vi "Register Message Metadata.vi"(8 "error in (no error)":errorcluster, 10 "Messages":T2[](array[typedef]), 11 "gRPCid":T1) -> (0 "error out":errorcluster, 3 "gRPCid":T1)   [LabVIEW 2020, in "helloWServer.lvlib" / "gprc-lvsupport.lvlib"]
uses:
  gprc-lvsupport.lvlib
  typeDefs/Message Metadata.ctl
  typeDefs/Message Element Metadata.ctl
  typeDefs/Message Element Type.ctl
  typeDefs/grpcId.ctl
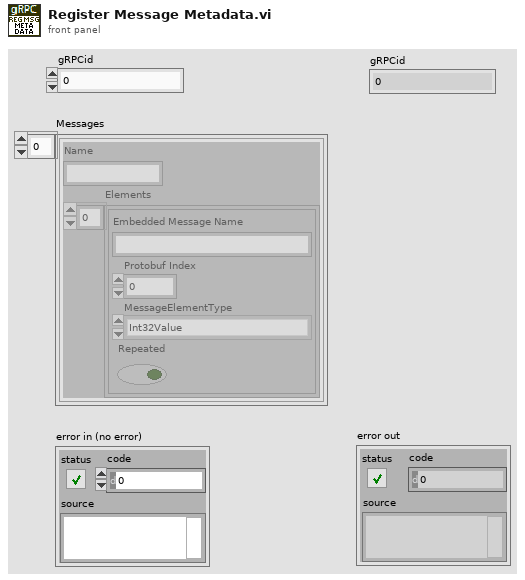
[diagram p1: front panel]
types:
  T1 = typedef "helloWServer.lvlib/gprc-lvsupport.lvlib/grpcId.ctl" = u64
  T2 = typedef "helloWServer.lvlib/gprc-lvsupport.lvlib/Message Metadata.ctl" = cluster{"Name":string, "Elements":T3[]}
  T3 = typedef "helloWServer.lvlib/gprc-lvsupport.lvlib/Message Element Metadata.ctl" = cluster{"Embedded Message Name":string, "Protobuf Index":i32, "MessageElementType":T4, "Repeated":bool}
  T4 = typedef "helloWServer.lvlib/gprc-lvsupport.lvlib/Message Element Type.ctl" = enum32{"Int32Value", "FloatValue", "DoubleValue", "BoolValue", "StringValue", "MessageValue", "Int64Value", "UInt32Value", "UInt64Value", "EnumValue"}
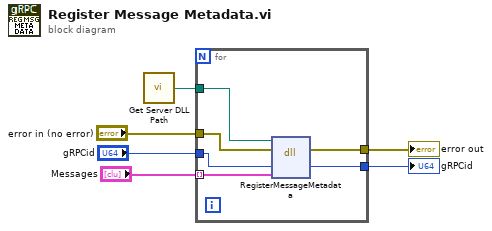
[diagram p0: block diagram]
diagram:
  n1 = call "Get Server DLL Path.vi"() -> ("Server dll path"=w1:path)
  n2 = for {
    tunnel: "Messages" -> [w12] mode=indexing
    tunnel: "gRPCid" -> [w11]
    tunnel: "error in (no error)" -> [w10]
    tunnel: [w9] -> w3
    tunnel: [w8] -> w2
    tunnel: w1 -> [w7]
    n3 = dll-call lib="C:/Users/XEnderMD/Desktop/LV gRPC/labview source/gRPC interface/dlls/labview_grpc_server.dll" fn="RegisterMessageMetadata"(path in=w7, error in=w10, "serverId"=w11, "metadata"=w12) -> (error out=w9:errorcluster, "serverId"=w8:T1)  [unwired: 3 in, 1 out]
  }
  "error out" <- w3
  "gRPCid" <- w2
